vi "liberaToCmd.vi"(4 "Set Environment":T1, 5 "value":string, 6 "loops":i32=1, 7 "acquire time":u32, 8 "samples":u32=1, 9 "triggered":bool, 10 "decimated":bool, 11 "cmd":T2(ring)=enum."acquireStream") -> (0 "jsonargs":string, 3 "cmd":string)   [LabVIEW 2014]
uses:
  libera_env.ctl
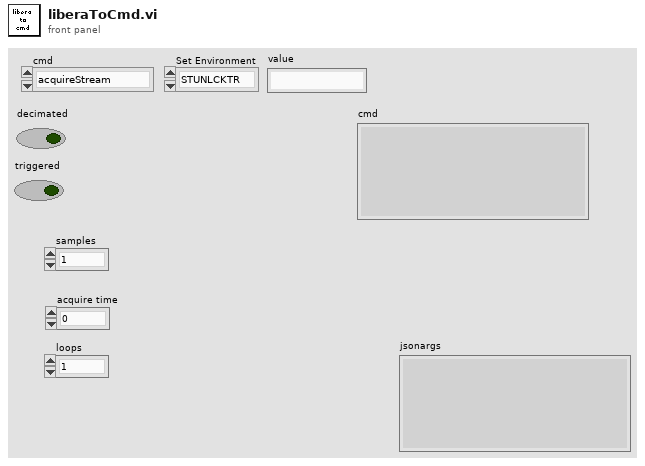
[diagram p1: front panel]
types:
  T1 = typedef "libera_env.ctl" = enum16{"STUNLCKTR", "TRIGMODE", "MTSYNCIN", "MTUNLCKTR", "MTNCOSHFT", "MTVCXOFFS", "POLYPHASE_FIR", "NOTCH2", "NOTCH1", "DDC_MAFDELAY", "DDC_MAFLENGTH", "SWDELAY", "EXTSWITCH", "TRIGDELAY", "PMDEC", "PMOFFSET", "ILKSTATUS", "ILK", "DSC", "AGC", "GAIN", "SWITCH", "QOFFSET", "YOFFSET", "XOFFSET", "KY", "KX"}
  T2 = enum16{"setEnv", "stopAcquire", "setTime", "acquireAVG", "acquireADCSP", "acquireADCCW", "acquireStream", "acquireDD"}
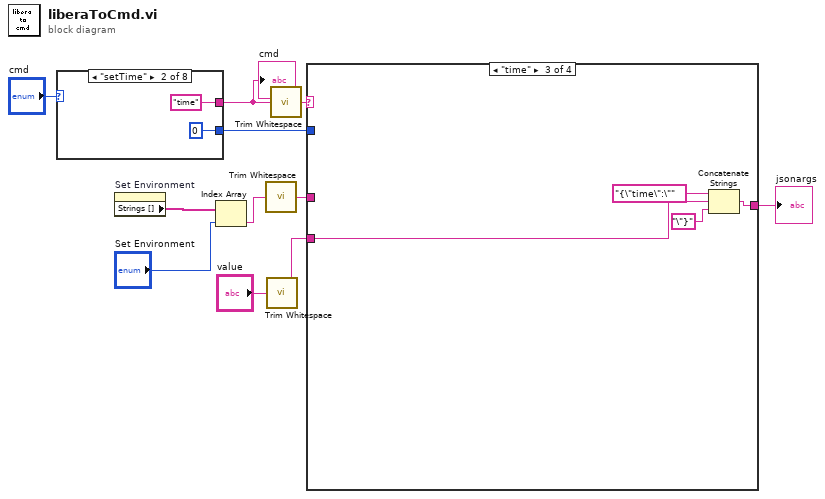
[diagram p0: block diagram]
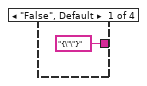
[diagram p2: hidden frame]
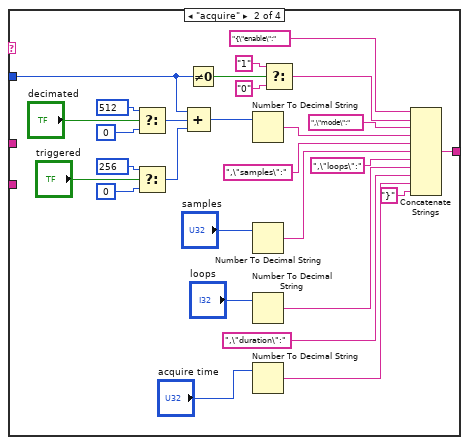
[diagram p3: hidden frame]
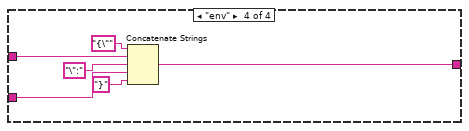
[diagram p4: hidden frame]
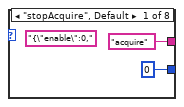
[diagram p5: hidden frame]
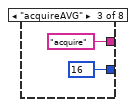
[diagram p6: hidden frame]
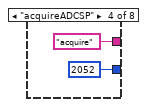
[diagram p7: hidden frame]
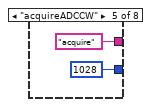
[diagram p8: hidden frame]
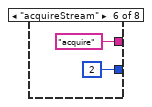
[diagram p9: hidden frame]
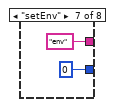
[diagram p10: hidden frame]
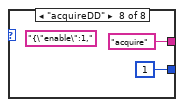
[diagram p11: hidden frame]
diagram:
  n1 = case shown="\"setTime\"" "cmd" {
    tunnel: ["acquire" "time" "acquire" "acquire" "acquire" "acquire" "env" "acquire"] -> w9
    tunnel: [u32 0 ("f") u32 0 ("f") u32 16 u32 2052 u32 1028 u32 2 u32 0 u32 1] -> w8
    frame "stopAcquire", Default {
      (unwired) "{\"enable\":0,"
    }
    frame "setTime" {
    }
    frame "acquireAVG" {
    }
    frame "acquireADCSP" {
    }
    frame "acquireADCCW" {
    }
    frame "acquireStream" {
    }
    frame "setEnv" {
    }
    frame "acquireDD" {
      (unwired) "{\"enable\":1,"
    }
  }
  "cmd" <- w9
  n2 = property on="Set Environment" class="Enum (strict)"() -> ("Strings []"=w7:string[])  [unwired: 2 in, 2 out]
  n3 = Index Array(array=w7, index="Set Environment") -> (element=w5:string)
  n4 = call <vilib>:"Trim Whitespace.vi"("string"=w5) -> ("trimmed string"=w1:string)  [unwired: 1 in]
  n5 = call <vilib>:"Trim Whitespace.vi"("string"="value") -> ("trimmed string"=w3:string)  [unwired: 1 in]
  n6 = call <vilib>:"Trim Whitespace.vi"("string"=w9) -> ("trimmed string"=w2:string)  [unwired: 1 in]
  n7 = case shown="\"time\"" w2 {
    tunnel: ["{\"\"}" w43 w57 w61] -> w10
    tunnel: w8 -> [_ w33 _ _]
    tunnel: w1 -> [_ _ _ w65]
    tunnel: w3 -> [_ _ w59 w63]
    frame "False", Default {
    }
    frame "acquire" {
      n8 = Select(t=u32 512, s="decimated", f=u32 0) -> (s? t:f=w37:u32)
      n9 = Select(t=u32 256, s="triggered", f=u32 0) -> (s? t:f=w36:u32)
      n10 = Not Equal To 0?(x=w33) -> (x != 0?=w32:bool)
      n11 = Compound Arithmetic op=ADD(w33, w37, w36) -> (w56:u32)
      n12 = Number To Decimal String(number=w56) -> (decimal integer string=w54:string)  [unwired: 1 in]
      n13 = Number To Decimal String(number="samples") -> (decimal integer string=w51:string)  [unwired: 1 in]
      n14 = Number To Decimal String(number="loops") -> (decimal integer string=w48:string)  [unwired: 1 in]
      n15 = Number To Decimal String(number="acquire time") -> (decimal integer string=w45:string)  [unwired: 1 in]
      n16 = Select(t="1", s=w32, f="0") -> (s? t:f=w29:string)
      n17 = Concatenate Strings("{\"enable\":", w29, ",\"mode\":" ("string"), w54, ",\"samples\":" ("string"), w51, ",\"loops\":" ("string"), w48, ",\"duration\":" ("string"), w45, "}" ("string")) -> (w43:string)
    }
    frame "time" {
      n18 = Concatenate Strings("{\"time\":\"" ("string"), w59, "\"}" ("string")) -> (w57:string)
    }
    frame "env" {
      n19 = Concatenate Strings("{\"" ("string"), w65, "\":" ("string"), w63, "}" ("string")) -> (w61:string)
    }
  }
  "jsonargs" <- w10
